vi "createDirectory.vi"(8 "error in (no error)":errorcluster, 10 "newDirectoryPath":path, 11 "Directory in":refnum<class "Directory.lvclass">) -> (0 "error out":errorcluster, 2 "newDirectoryPath 2":path, 3 "Directory out":refnum<class "Directory.lvclass">)   [LabVIEW 2012, in "Directory.lvclass"]
uses:
  Directory.lvclass
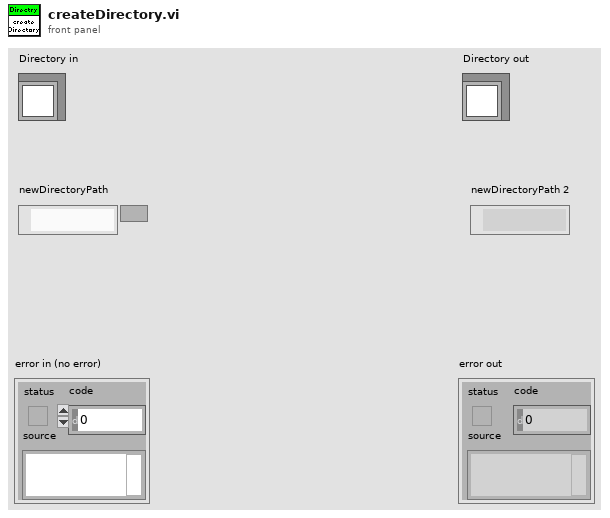
[diagram p1: front panel]
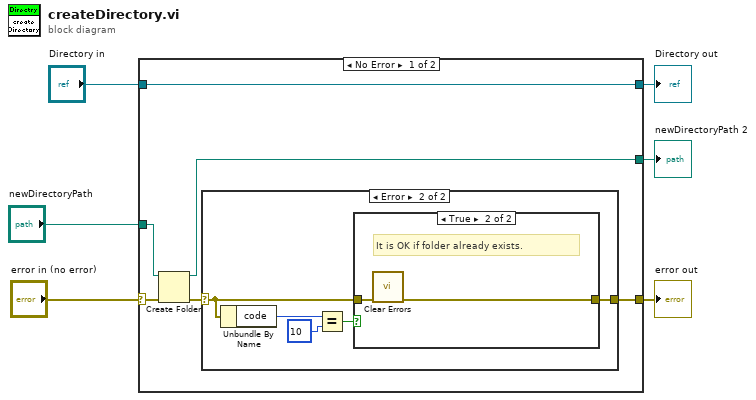
[diagram p0: block diagram]
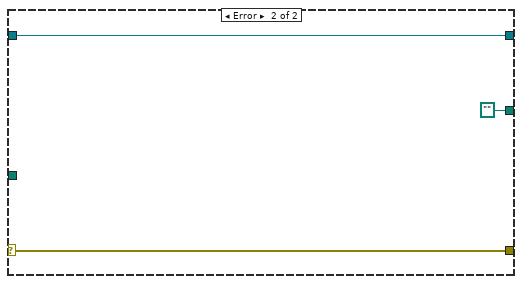
[diagram p4: hidden frame]
diagram:
  n1 = case shown="No Error" "error in (no error)" {
    selector: "error in (no error)" -> [w8 w24]
    tunnel: [w7 w24] -> w5
    tunnel: [w12 w23] -> w3
    tunnel: "Directory in" -> [w12 w23]
    tunnel: "newDirectoryPath" -> [w10 _]
    tunnel: [w9 path ""] -> w1
    frame No Error {
      n2 = Create Folder(path (use dialog)=w10, error in=w8) -> (created path=w9:path, error out=w11:errorcluster)  [unwired: 1 in, 1 out]
      n3 = case shown="Error" w11 {
        selector: w11 -> [w13 w16]
        tunnel: [w13 w15] -> w7
        frame No Error {
        }
        frame Error {
          n4 = Unbundle By Name(w16) -> ("code"=w18:i32)
          n5 = Equal?(x=w18, y=10) -> (x = y?=w14:bool)
          n6 = case shown="True" w14 {
            tunnel: w16 -> [w19 w21]
            tunnel: [w19 w20] -> w15
            frame False {
            }
            frame True {
              # "It is OK if folder already exists."
              n7 = call <vilib>:"Clear Errors.vi"("error in (no error)"=w21) -> ("error out"=w20:errorcluster)  [unwired: 6 in]
            }
          }
        }
      }
    }
    frame Error {
    }
  }
  "error out" <- w5
  "Directory out" <- w3
  "newDirectoryPath 2" <- w1
